vi "Constants.vi"() -> ()   [LabVIEW 2019, in "Profile Interpolation Shared.lvlib"]
doc: "Use this Global VI to access the GUIDs assigned to the page resources of the Custom Device."
uses:
  Profile Interpolation Shared.lvlib
panel:
  in  "Tab Control":enum32{"GUIDS", "Constants", "Properties"}(tab)
  in  "NoUnit.IN.CH.GUID":string="d5cc2b17-ef30-46e8-a564-131f4d83aa87"
  in  "Outputs.SEC.GUID":string="151e1bc7-0423-44e0-a438-2cf79b778960"
  in  "Inputs.SEC.GUID":string="c760ddfa-25b1-4f1f-b6f6-158bab5c488c"
  in  "NoUnit.OUT.CH.GUID":string="03d25316-c984-40a2-b7a5-299d4ae45b3d"
  in  "ProfileSelect.IN.CH.GUID":string="dc3d6906-b701-406a-8340-ad1fba4aee4f"
  in  "Unit.OUT.CH.GUID":string="a5671c29-93a6-4bf9-bfe3-9d14a3bb9949"
  in  "Table.SEC.GUID":string="255732fb-9748-4748-9b6b-077d2de97b58"
  in  "StatusChannels.SEC.GUID":string="0f474b91-5aac-4f3e-bdee-8596ccf1b61e"
  in  "Unit.IN.CH.GUID":string="ae661831-c210-403b-b869-35458f2e7103"
  in  "StatusChannels.OUT.CH.GUID":string="597327b9-7b32-41b7-8f6b-6f91baffe172"
  in  "Profile Interpolation Custom Device GUID":string="dc28dedc-b51d-49af-b49d-2a803ac116dd"
  in  "YMeasured.CH.NAME":string="Measured"
  in  "Setpoint.CH.NAME":string="Setpoint"
  in  "XMeasured.CH.NAME":string="Measured"
  in  "UpperLimit.CH.NAME":string="Upper Limit"
  in  "LowerLimit.CH.NAME":string="Lower Limit"
  in  "LimitViolation.CH.NAME":string="Limit Violation"
  in  "LimitEnable.CH.NAME":string="Limit Enable"
  in  "Outputs.SEC.NAME":string="Outputs"
  in  "Inputs.SEC.NAME":string="Inputs"
  in  "TableLength.CH.NAME":string="Table Length"
  in  "ProfileCount.CH.NAME":string="Profile Count"
  in  "ProfileSelect.CH.NAME":string="Profile Select"
  in  "StatusChannels.SEC.NAME":string="Status Channels"
  in  "Table.SEC.NAME":string="Table"
  in  "Interpolation.File.Target":string="Interpolation.File.Target"
  in  "Create.Limit.Channels":string="Profiles"
  in  "Interpolation.File.Host":string="Interpolation.File.Host"
  in  "Compiled.Settings":string="Compiled.Settings"
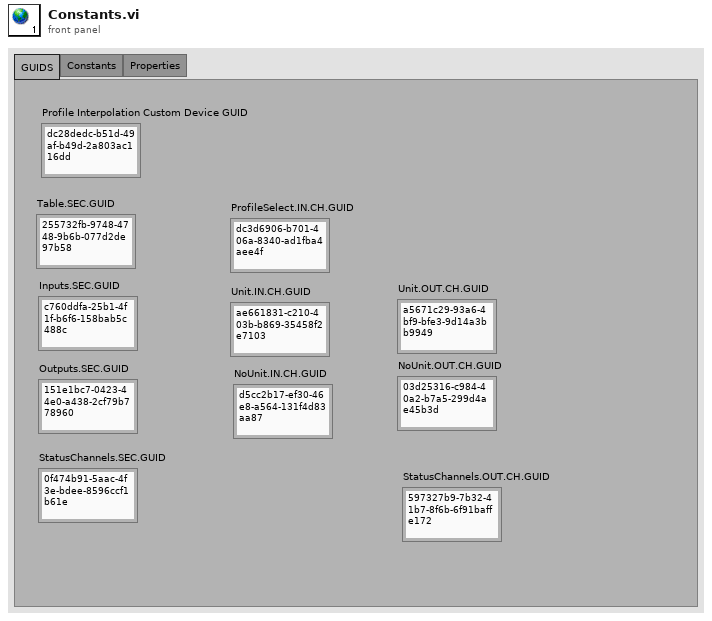
[diagram p1: front panel]
diagram:
